vi "F020_digtal_get.vi"(8 "error in":errorcluster, 10 "ADDRESS":u8=170, 11 "COM in":string="COM2") -> (0 "error out":errorcluster={"status"=TRUE, "code"=-1073807343, "source"=""}, 2 "DINPORTSx6+StatusRegister":u8[](array[numeric]) format="%.0x", 3 "COM out":string="COM4", 4 "DIGITAL_IO":T1={"DIG_PORT_0 [0..7] (P4)"=[FALSE, FALSE, FALSE, FALSE, FALSE, FALSE, FALSE, FALSE], "DIG_PORT_1 [8..15] (P5)"=[FALSE, FALSE, FALSE, FALSE, FALSE, FALSE, FALSE, FALSE], "DIG_PORT_2 [16..23]  (P3)"=[TRUE, TRUE, FALSE, TRUE, FALSE, TRUE, FALSE, TRUE], "DIG_PORT_3  [23..31]  (P2)"=[TRUE, TRUE, FALSE, TRUE, FALSE, TRUE, FALSE, TRUE], "DIG_PORT_4   [32..39]  (P6)"=[FALSE, FALSE, FALSE, FALSE, FALSE, FALSE, FALSE, FALSE], "DIG_PORT_5  [40..47]  (P7)"=[FALSE, FALSE, FALSE, FALSE, FALSE, FALSE, FALSE, FALSE]}, 6 "Digital Pins Index":bool[](array[boolean]))   [LabVIEW 2016]
doc: "This example performs a serial port write and a serial port read. The parameters set for the serial port must match the parameters of the connected instrument or device. The VISA Configure Serial Port VI sets the configuration parameters. The front panel displays the controls used to configure the basic parameters, such as baud rate, data bits, and parity. The VI passes the VISA resource name to other VIs that perform operations on that VISA resource. The VISA Write function sends a command to the serial device and the VISA Read function returns data based on the command. The VISA Close function then closes the reference to the serial device. It is important to close the reference; otherwise, further communication through that port might not be possible."
panel:
  # "loopback: <xxAABB>\nwr_dout:   <xxAA11aabbccdd> aa=ch, bb=val, ccdd=timeout[sec]\nrd_ain:      <xxAA13aa> -> {qqww}"
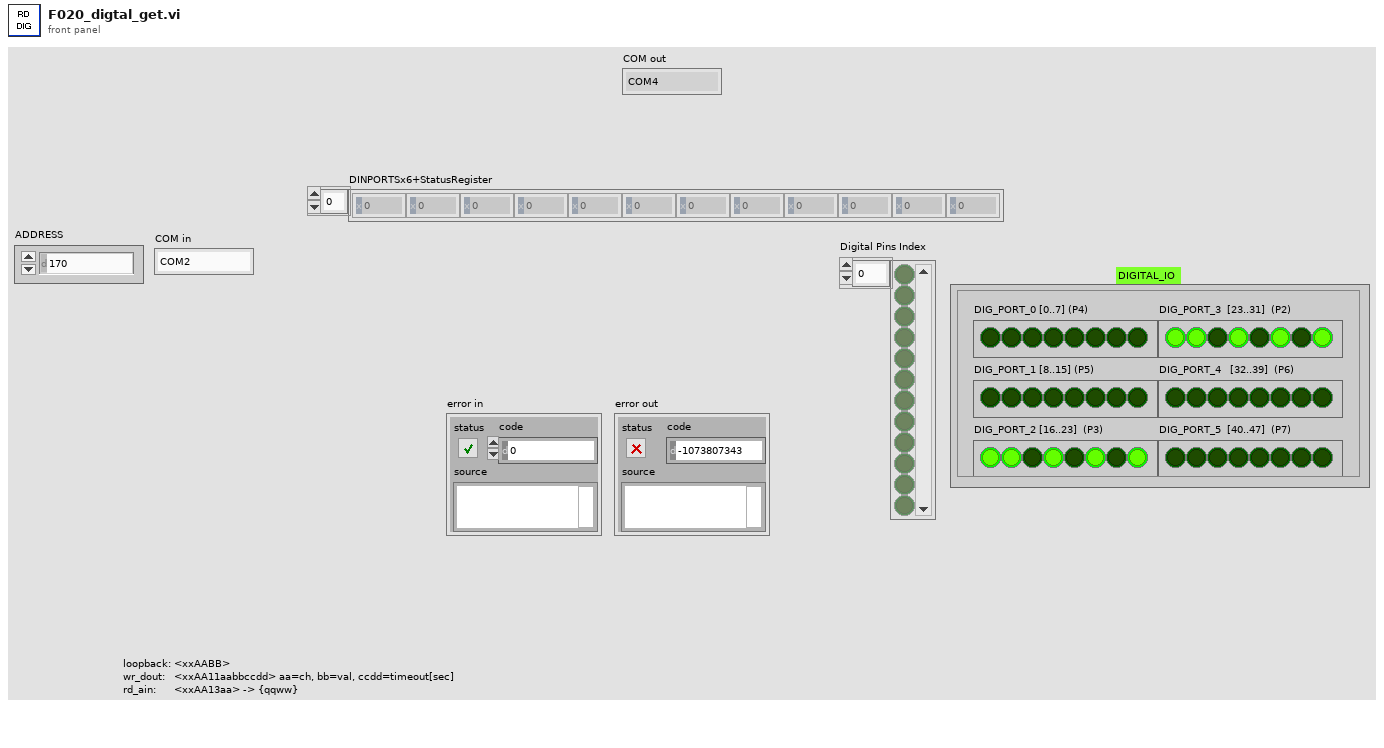
[diagram p1: front panel]
types:
  T1 = cluster{"DIG_PORT_0 [0..7] (P4)":bool[], "DIG_PORT_1 [8..15] (P5)":bool[], "DIG_PORT_2 [16..23]  (P3)":bool[], "DIG_PORT_3  [23..31]  (P2)":bool[], "DIG_PORT_4   [32..39]  (P6)":bool[], "DIG_PORT_5  [40..47]  (P7)":bool[]}
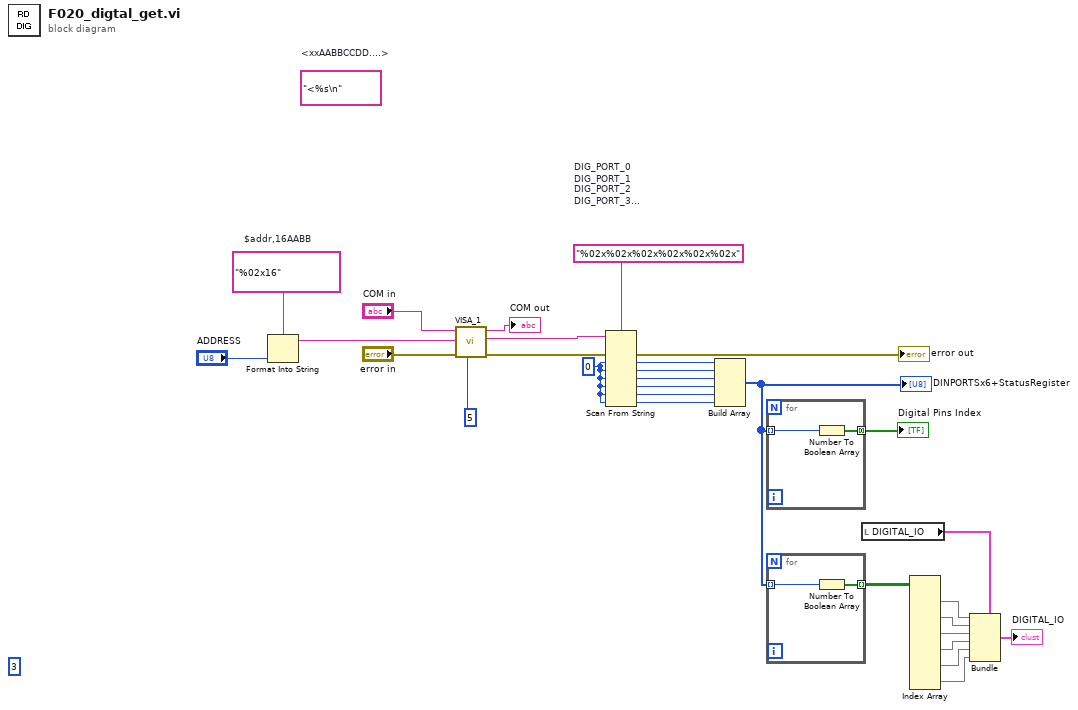
[diagram p0: block diagram]
diagram:
  w18 = u8 0 ("default value 1")
  w25 = "%02x%02x%02x%02x%02x%02x"  # DIG_PORT_0 DIG_PORT_1 DIG_PORT_2 DIG_PORT_3 DIG_PORT_4 DIG_PORT_5 STATUS_REGISTER
  (unwired) u32 3 ("delay before read (ms)")
  w26 = "%02x16"  # $addr,16AABB
  (unwired) "<%s\n"  # <xxAABBCCDD....>
  n1 = Format Into String(format string=w26, "ADDRESS") -> (resulting string=w1:string)  [unwired: 2 in, 1 out]
  n2 = call "VISA_1.vi"("delay[ms]"=u32 5, "error in"="error in", "wr_buf"=w1, "COM in"="COM in") -> ("error out"=w21:errorcluster, "rx_buf"=w5:string, "COM out"=→"COM out":string)  [unwired: 4 in, 1 out]
  n3 = Scan From String(format string=w25, input string=w5, error in=w21, default 1=w18, default 2=w18, default 3=w18, default 4=w18, default 5=w18, default 6=w18) -> (error out=→"error out":errorcluster, output 1=w24:u8, output 2=w23:u8, output 3=w22:u8, output 4=w20:u8, output 5=w19:u8, output 6=w17:u8)  [unwired: 1 in, 2 out]
  n4 = Build Array(w24, w23, w22, w20, w19, w17) -> (w8:u8[])
  "DINPORTSx6+StatusRegister" <- w8
  n5 = for {
    tunnel: w8 -> [w31] mode=indexing
    tunnel: [w30] -> w6 mode=concatenating
    n6 = Number To Boolean Array(number=w31) -> (Boolean array=w30:bool[])
  }
  "Digital Pins Index" <- w6
  n7 = for {
    tunnel: w8 -> [w33] mode=indexing
    tunnel: [w32] -> w15 mode=indexing
    n8 = Number To Boolean Array(number=w33) -> (Boolean array=w32:bool[])
  }
  n9 = local read "DIGITAL_IO"() -> (w7:T1)
  n10 = Index Array(array=w15) -> (element #1=w14:bool[], element #2=w13:bool[], element #3=w12:bool[], element #4=w11:bool[], element #5=w10:bool[], element #6=w9:bool[])  [unwired: 12 in]
  n11 = Bundle(cluster=w7, "DIG_PORT_0 [0..7] (P4)"=w14, "DIG_PORT_1 [8..15] (P5)"=w13, "DIG_PORT_2 [16..23]  (P3)"=w12, "DIG_PORT_3  [23..31]  (P2)"=w11, "DIG_PORT_4   [32..39]  (P6)"=w10, "DIG_PORT_5  [40..47]  (P7)"=w9) -> (→"DIGITAL_IO":T1)
